vi "Fetch Elog Array.vi"(8 "error in":errorcluster, 10 "Type":u16(ring) items=["Data"], 11 "VISA resource name":refnum<visa-resource-name>) -> (0 "error out":errorcluster, 2 "Value":string, 3 "VISA resource name out":refnum<visa-resource-name>)   [LabVIEW 2015, in "IT-M3900C.lvlib"]
doc: "This command is used to query the voltage and current values of corresponding data records.\n<b>Type</b>\nData：Query the average value of voltage and current."
uses:
  <instrlib>/IT-M3900C/IT-M3900C.lvlib
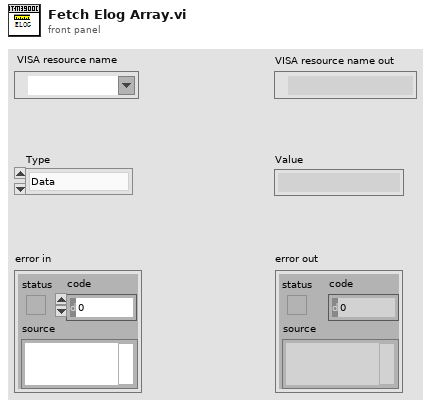
[diagram p1: front panel]
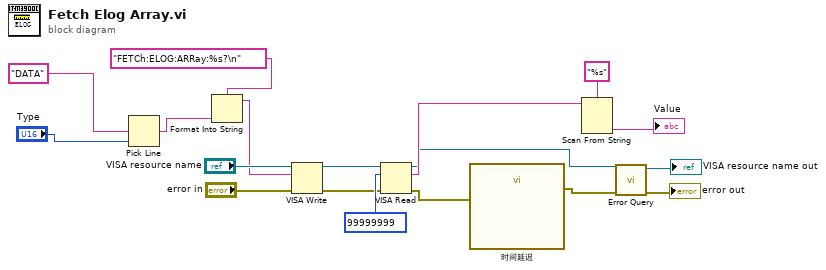
[diagram p0: block diagram]
diagram:
  n1 = Pick Line(multi-line string="DATA" ("多行字符串"), line index="Type") -> (output string=w7:string)  [unwired: 1 in]
  n2 = Format Into String(format string="FETCh:ELOG:ARRay:%s?\n", w7) -> (resulting string=w4:string)  [unwired: 2 in, 1 out]
  n3 = VISA Write(VISA resource name="VISA resource name", write buffer=w4, error in (no error)="error in") -> (VISA resource name out=w10:refnum<visa-resource-name>, error out=w9:errorcluster)  [unwired: 1 out]
  n4 = VISA Read(VISA resource name=w10, byte count=99999999, error in (no error)=w9) -> (VISA resource name out=w3:refnum<visa-resource-name>, read buffer=w16:string, error out=w2:errorcluster)  [unwired: 1 out]
  n5 = call "时间延迟"("error in (no error)"=w2) -> ("error out"=w1:errorcluster)  [unwired: 10 in]
  n6 = Scan From String(format string="%s", input string=w16) -> (output 1=→"Value":string)  [unwired: 3 in, 3 out]
  n7 = call <instrlib>:"Error Query.vi"("error in"=w1, "VISA resource name"=w3) -> ("error out"=→"error out":errorcluster, "VISA resource name out"=→"VISA resource name out":refnum<visa-resource-name>)  [unwired: 6 in, 2 out]
